vi "Convert_JSON_to_allChannelProperties.vi"(8 "error in (no error)":errorcluster, 11 "<JSON>":string) -> (0 "error out":errorcluster, 3 "allChannelProperties":T1 {"channel" min=1 max=8 step=1})   [LabVIEW 2019, in "Inst.Krohn-Hite-7008.lvclass"]
uses:
  Inst.Krohn-Hite-7008.lvclass
  KH7008/typedefs/allChannelProperties--Array.ctl
  KH7008/typedefs/channelProperties--Cluster.ctl
  KH7008/typedefs/channel--numeric.ctl
  KH7008/typedefs/gain--enum.ctl
  KH7008/typedefs/Input--Enum.ctl
  KH7008/typedefs/shunt--enum.ctl
  KH7008/typedefs/couple--Enum.ctl
  KH7008/typedefs/Filter--Enum.ctl
  <vilib>/regexp/Match Regular Expression.xnode
  KH7008/KH7008.lvlib
  <vilib>/JDP Science/JSONtext/JSONtext.lvlib
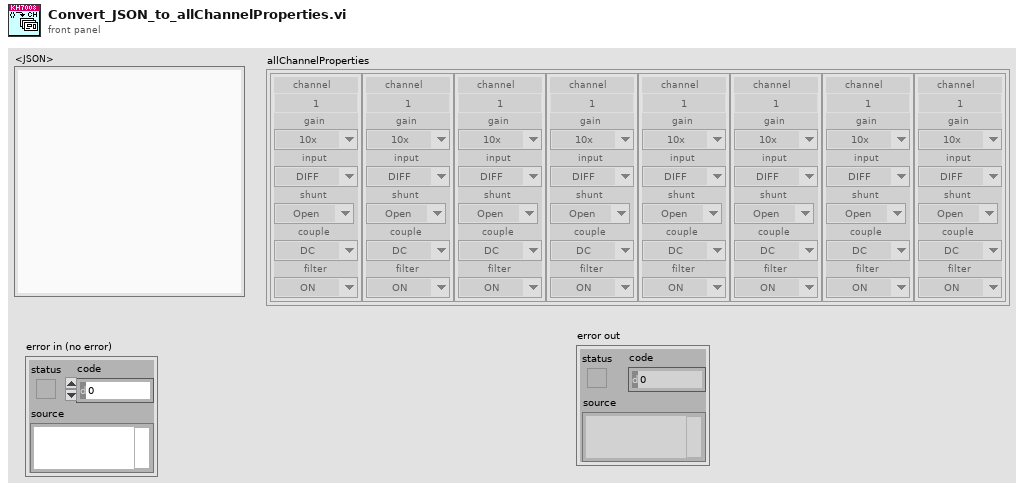
[diagram p1: front panel]
types:
  T1 = typedef "KH7008.lvlib/allChannelProperties--Array.ctl" = T2[]
  T2 = typedef "KH7008.lvlib/channelProperties--Cluster.ctl" = cluster{"channel":T3, "gain":T4, "input":T5, "shunt":T6, "couple":T7, "filter":T8}
  T3 = typedef "KH7008.lvlib/channel--numeric.ctl" = u16
  T4 = typedef "KH7008.lvlib/gain--enum.ctl" = enum16{"1x", "10x", "100x", "1000x"}
  T5 = typedef "KH7008.lvlib/input--enum.ctl" = enum16{"OFF", "SE+", "SE-", "DIFF"}
  T6 = typedef "KH7008.lvlib/shunt--enum.ctl" = enum16{"Open", "50", "500", "5k", "50k", "10M"}
  T7 = typedef "KH7008.lvlib/couple--enum.ctl" = enum16{"AC", "DC"}
  T8 = typedef "KH7008.lvlib/filter--enum.ctl" = enum16{"OFF", "ON"}
  T9 = typedef "JSONtext.lvlib/JSON Value Type.ctl" = enum16{"Not a JSON Value", "JSON Object", "JSON Array", "String", "Number", "true", "false", "null"}
  T10 = typedef "KH7008.lvlib/Input--Enum.ctl" = enum16{"OFF", "SE+", "SE-", "DIFF"}
  T11 = typedef "KH7008.lvlib/couple--Enum.ctl" = enum16{"AC", "DC"}
  T12 = typedef "KH7008.lvlib/Filter--Enum.ctl" = enum16{"OFF", "ON"}
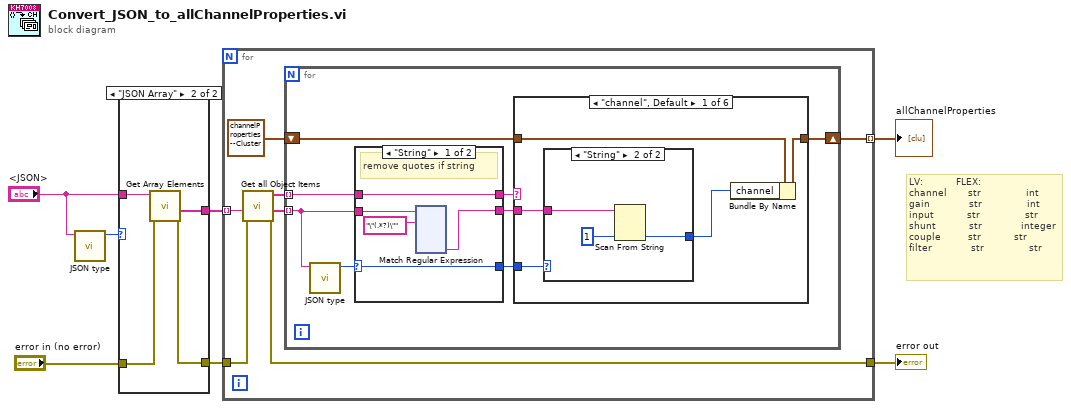
[diagram p0: block diagram]
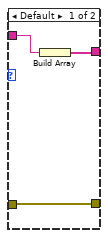
[diagram p2: hidden frame]
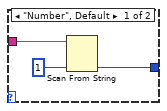
[diagram p4: hidden frame]
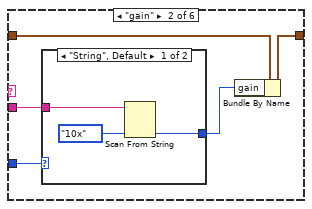
[diagram p5: hidden frame]
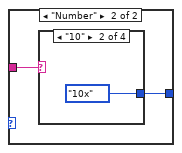
[diagram p6: hidden frame]
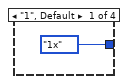
[diagram p7: hidden frame]
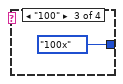
[diagram p8: hidden frame]
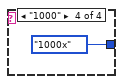
[diagram p9: hidden frame]
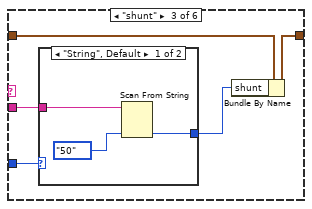
[diagram p10: hidden frame]
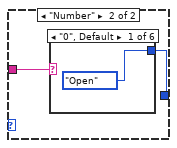
[diagram p11: hidden frame]
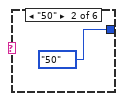
[diagram p12: hidden frame]
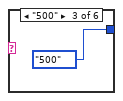
[diagram p13: hidden frame]
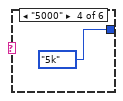
[diagram p14: hidden frame]
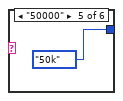
[diagram p15: hidden frame]
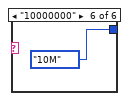
[diagram p16: hidden frame]
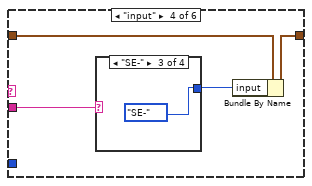
[diagram p17: hidden frame]
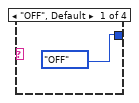
[diagram p18: hidden frame]
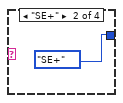
[diagram p19: hidden frame]
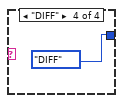
[diagram p20: hidden frame]
diagram:
  # "LV:           FLEX:\nchannel       str               int\ngain             str               int\ninput           str               str\nshunt           str             integer\ncouple         str           str\nfilter             str               str"
  n1 = call <vilib>:"JSON type.vi"("JSON"="<JSON>") -> ("JSON Value Type"=w1:T9)  [unwired: 9 in, 1 out]
  n2 = case shown="\"JSON Array\"" w1 {
    tunnel: [w9 w14] -> w6
    tunnel: "error in (no error)" -> [w8 w13]
    tunnel: [w8 w12] -> w4
    tunnel: "<JSON>" -> [w10 w11]
    frame Default {
      n3 = Build Array(w10) -> (w9:string[])
    }
    frame "JSON Array" {
      n4 = call <vilib>:"Get Array Elements.vi"("error in (no error)"=w13, "JSON"=w11) -> ("error out"=w12:errorcluster, "<JSON>"=w14:string[])  [unwired: 7 in, 1 out]
    }
  }
  n5 = for {
    tunnel: w6 -> [w19] mode=indexing
    tunnel: [w20] -> w7 mode=indexing
    tunnel: w4 -> [w16]
    tunnel: [w15] -> w3
    n6 = call <vilib>:"Get all Object Items.vi"("error in (no error)"=w16, "JSON"=w19) -> ("error out"=w15:errorcluster, "<JSON>"=w17:string[], "Item Names"=w18:string[])  [unwired: 6 in, 1 out]
    n7 = for {
      tunnel: w18 -> [w22] mode=indexing
      shift-right: [w28] -> w20
      shift-left: T2 {"channel"=1, "gain"=enum."10x", "input"=enum."DIFF", "shunt"=enum."Open", "couple"=enum."DC", "filter"=enum."ON"} ("channelProperties") -> [w29]
      tunnel: w17 -> [w26] mode=indexing
      n8 = call <vilib>:"JSON type.vi"("JSON"=w26) -> ("JSON Value Type"=w25:T9)  [unwired: 9 in, 1 out]
      n9 = case shown="\"String\"" w25 {
        selector: w25 -> [w34 w152]
        tunnel: [w31 w153] -> w27
        tunnel: w26 -> [w32 w153]
        tunnel: [w34 w152] -> w24
        tunnel: [w30 w151] -> w23
        tunnel: w22 -> [w30 w151]
        frame "String" {
          # "remove quotes if string"
          n10 = xnode "Match Regular Expression"("input string"=w32, "regular expression"="\"(.*?)\"") -> ("submatch 1"=w31:string)  [unwired: 4 in, 5 out]
        }
        frame "Number", Default {
        }
      }
      n11 = case shown="\"channel\", Default" w23 {
        tunnel: w29 -> [w157 w168 w182 w197 w205 w211]
        tunnel: [w158 w169 w183 w198 w206 w212] -> w28
        tunnel: w27 -> [w155 w166 w181 w195 w203 w209]
        tunnel: w24 -> [w154 w165 w180 _ _ _]
        frame "channel", Default {
          n12 = case shown="\"String\"" w154 {
            tunnel: [w159 w162] -> w156
            tunnel: w155 -> [w161 w164]
            frame "Number", Default {
              n13 = Scan From String(input string=w161, default 1=T3 1 ("channel")) -> (output 1=w159:T3)  [unwired: 3 in, 3 out]
            }
            frame "String" {
              n14 = Scan From String(input string=w164, default 1=T3 1 ("channel")) -> (output 1=w162:T3)  [unwired: 3 in, 3 out]
            }
          }
          n15 = Bundle By Name(cluster=w157, "channel"=w156) -> (w158:T2)
        }
        frame "gain" {
          n16 = case shown="\"String\", Default" w165 {
            tunnel: [w171 w174] -> w167
            tunnel: w166 -> [w172 w173]
            frame "String", Default {
              n17 = Scan From String(input string=w172, default 1=gain--enum."10x" ("gain")) -> (output 1=w171:T4)  [unwired: 3 in, 3 out]
            }
            frame "Number" {
              n18 = case shown="\"10\"" w173 {
                tunnel: [gain--enum."1x" ("gain") gain--enum."10x" ("gain") gain--enum."100x" ("gain") gain--enum."1000x" ("gain")] -> w174
                frame "1", Default {
                }
                frame "10" {
                }
                frame "100" {
                }
                frame "1000" {
                }
              }
            }
          }
          n19 = Bundle By Name(cluster=w168, "gain"=w167) -> (w169:T2)
        }
        frame "shunt" {
          n20 = case shown="\"String\", Default" w180 {
            tunnel: [w184 w188] -> w179
            tunnel: w181 -> [w186 w187]
            frame "String", Default {
              n21 = Scan From String(input string=w186, default 1=shunt--enum."50" ("shunt")) -> (output 1=w184:T6)  [unwired: 3 in, 3 out]
            }
            frame "Number" {
              n22 = case shown="\"0\", Default" w187 {
                tunnel: [shunt--enum."Open" ("shunt") shunt--enum."50" ("shunt") shunt--enum."500" ("shunt") shunt--enum."5k" ("shunt") shunt--enum."50k" ("shunt") shunt--enum."10M" ("shunt")] -> w188
                frame "0", Default {
                }
                frame "50" {
                }
                frame "500" {
                }
                frame "5000" {
                }
                frame "50000" {
                }
                frame "10000000" {
                }
              }
            }
          }
          n23 = Bundle By Name(cluster=w182, "shunt"=w179) -> (w183:T2)
        }
        frame "input" {
          n24 = case shown="\"SE-\"" w195 {
            tunnel: [Input--Enum."OFF" ("input") Input--Enum."SE+" ("input") Input--Enum."SE-" ("input") Input--Enum."DIFF" ("input")] -> w196
            frame "OFF", Default {
            }
            frame "SE+" {
            }
            frame "SE-" {
            }
            frame "DIFF" {
            }
          }
          n25 = Bundle By Name(cluster=w197, "input"=w196) -> (w198:T2)
        }
        frame "couple" {
          n26 = case shown="\"DC\"" w203 {
            tunnel: [couple--Enum."DC" ("couple") couple--Enum."AC" ("couple")] -> w204
            frame "DC" {
            }
            frame "AC", Default {
            }
          }
          n27 = Bundle By Name(cluster=w205, "couple"=w204) -> (w206:T2)
        }
        frame "filter" {
          n28 = case shown="\"OFF\", Default" w209 {
            tunnel: [Filter--Enum."OFF" ("filter") Filter--Enum."ON" ("filter")] -> w210
            frame "OFF", Default {
            }
            frame "ON" {
            }
          }
          n29 = Bundle By Name(cluster=w211, "filter"=w210) -> (w212:T2)
        }
      }
    }
  }
  "allChannelProperties" <- w7
  "error out" <- w3
